vi "Read XML_Parameters_Check File Against Schema.vi"(8 "error in (no error)":errorcluster, 10 "XML Schema File Path":path=path "E:/Ballard - Arinc-429 CD/Source/System Explorer/SubVIs/Parse XML Ballard/BTI.XSD", 11 "XML Configuration File Path":path=path "E:/Ballard - Arinc-429 CD/Example Database/Ballard/XML_000.XML") -> (0 "error IO":errorcluster, 3 "ValidateAgainstXMLSchema":bool)   [LabVIEW 2019, in "Ballard Arinc-429 System Explorer.lvlib"]
uses:
  Ballard Arinc-429 System Explorer.lvlib
  C:/Users/Localization Tester/Desktop/GIT/Ballard-Arinc-429-Custom-Device/Source/System Explorer/SubVIs/Parse Parameters File/Parameters_Arinc429_XML_Tools.dll
  Parameters_Arinc429_XML_Tools.dll
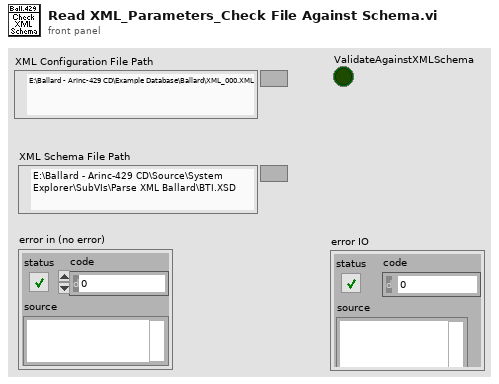
[diagram p1: front panel]
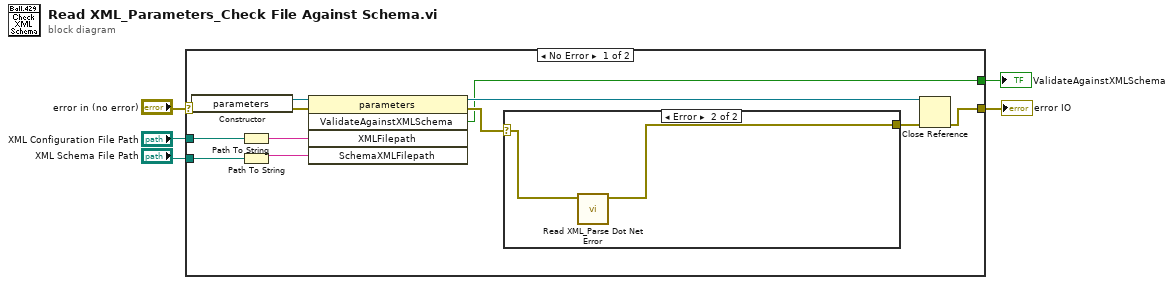
[diagram p0: block diagram]
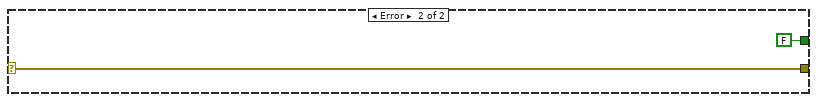
[diagram p3: hidden frame]
diagram:
  n1 = case shown="No Error" "error in (no error)" {
    selector: "error in (no error)" -> [w13 w22]
    tunnel: "XML Configuration File Path" -> [w17 _]
    tunnel: "XML Schema File Path" -> [w16 _]
    tunnel: [w14 w22] -> w2
    tunnel: [w6 FALSE ("ValidateAgainstXMLSchema")] -> w1
    frame No Error {
      n2 = constructor class="parameters"(error in=w13) -> (reference out=w12:refnum<k24>, error out=w11:errorcluster)  [unwired: 2 in, 1 out]
      n3 = Path To String(path=w17) -> (string=w10:string)
      n4 = Path To String(path=w16) -> (string=w9:string)
      n5 = invoke class="parameters" method="ValidateAgainstXMLSchema"(reference=w12, error in=w11, "XMLFilepath"=w10, "SchemaXMLFilepath"=w9) -> (reference out=w8:refnum<k24>, error out=w7:errorcluster, "ValidateAgainstXMLSchema"=w6:bool)  [unwired: 1 in, 2 out]
      n6 = case shown="Error" w7 {
        selector: w7 -> [w18 w20]
        tunnel: [w18 w19] -> w15
        frame No Error {
        }
        frame Error {
          n7 = call "Read XML_Parse Dot Net Error.vi"("error in (no error)"=w20) -> ("error out"=w19:errorcluster)  [unwired: 10 in]
        }
      }
      n8 = Close Reference(reference=w8, error in (no error)=w15) -> (error out=w14:errorcluster)
    }
    frame Error {
    }
  }
  "error IO" <- w2
  "ValidateAgainstXMLSchema" <- w1
